vi "Example Configuration.vi"() -> ()   [LabVIEW 2013]
uses:
  C:/tf/play/labview/Tinkerforge.dll
panel:
  in  "uid":string="6dKCNw"
  in  "port":i32=4223
  in  "host":string="localhost"
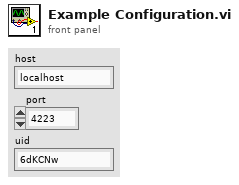
[diagram p1: front panel]
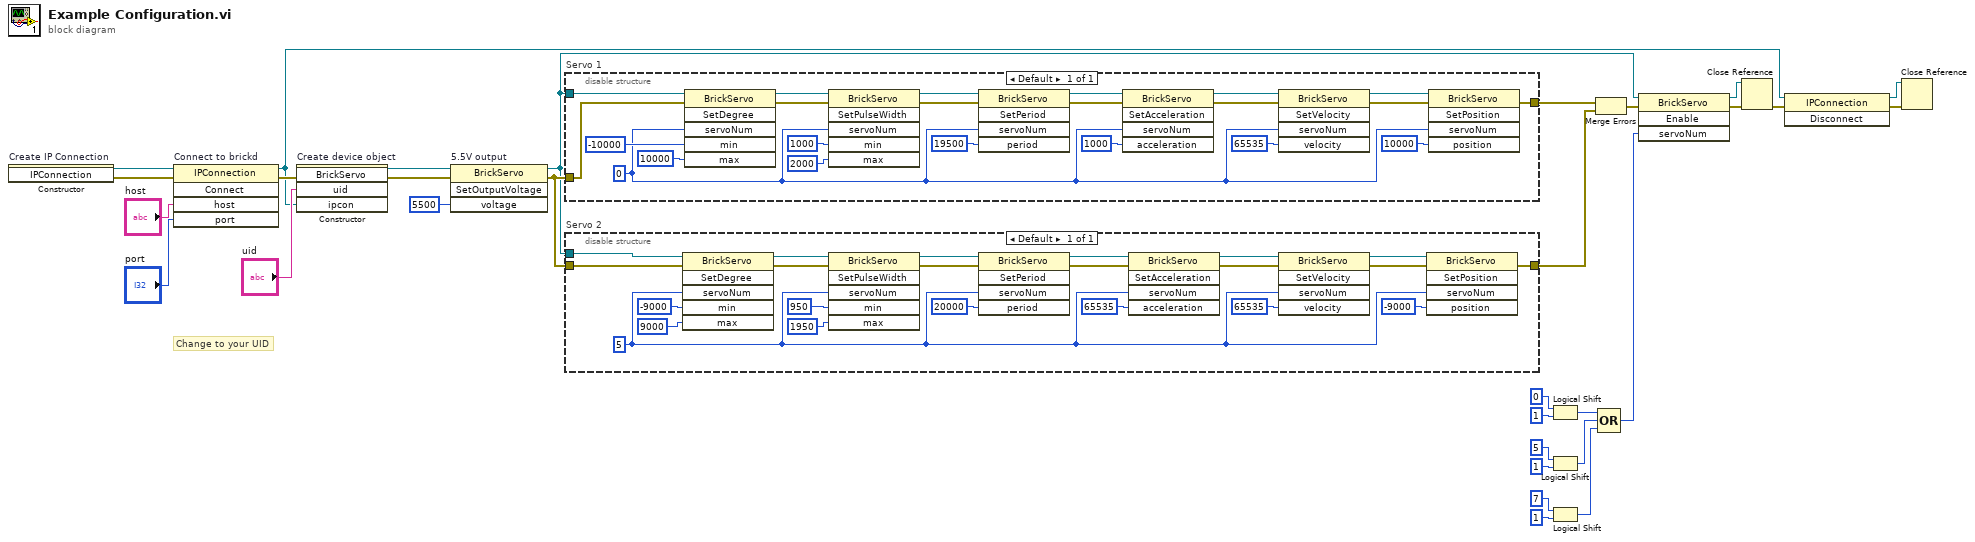
[diagram p0: block diagram]
diagram:
  # "Change to your UID"
  n1 = constructor on="Create IP Connection" class="IPConnection"() -> (reference out=w30:refnum<k24>, error out=w1:errorcluster)  [unwired: 3 in, 1 out]
  n2 = invoke on="Connect to brickd" class="IPConnection" method="Connect"(reference=w30, error in=w1, "host"="host", "port"="port") -> (reference out=w21:refnum<k24>, error out=w26:errorcluster)  [unwired: 1 in, 3 out]
  n3 = constructor on="Create device object" class="BrickServo"(error in=w26, "uid"="uid", "ipcon"=w21) -> (reference out=w24:refnum<k24>, error out=w25:errorcluster)  [unwired: 2 in, 3 out]
  n4 = invoke on="5.5V output" class="BrickServo" method="SetOutputVoltage"(reference=w24, error in=w25, "voltage"=5500 ("current")) -> (reference out=w15:refnum<k24>, error out=w18:errorcluster)  [unwired: 1 in, 2 out]
  n5 = disable-structure "Servo 1" shown="Default" {
    disable-tunnel: w15 -> [w50]
    disable-tunnel: w18 -> [w49]
    disable-tunnel: [w38] -> w16
    frame Enabled {
      w37 = u8 0 ("mode")
      n6 = invoke class="BrickServo" method="SetDegree"(reference=w50, error in=w49, "servoNum"=w37, "min"=i16 -10000, "max"=i16 10000) -> (reference out=w46:refnum<k24>, error out=w48:errorcluster)  [unwired: 1 in, 4 out]
      n7 = invoke class="BrickServo" method="SetPulseWidth"(reference=w46, error in=w48, "servoNum"=w37, "min"=1000, "max"=2000) -> (reference out=w45:refnum<k24>, error out=w47:errorcluster)  [unwired: 1 in, 4 out]
      n8 = invoke class="BrickServo" method="SetPeriod"(reference=w45, error in=w47, "servoNum"=w37, "period"=19500) -> (reference out=w43:refnum<k24>, error out=w44:errorcluster)  [unwired: 1 in, 3 out]
      n9 = invoke class="BrickServo" method="SetAcceleration"(reference=w43, error in=w44, "servoNum"=w37, "acceleration"=1000) -> (reference out=w41:refnum<k24>, error out=w42:errorcluster)  [unwired: 1 in, 3 out]
      n10 = invoke class="BrickServo" method="SetVelocity"(reference=w41, error in=w42, "servoNum"=w37, "velocity"=65535 ("acceleration")) -> (reference out=w39:refnum<k24>, error out=w40:errorcluster)  [unwired: 1 in, 3 out]
      n11 = invoke class="BrickServo" method="SetPosition"(reference=w39, error in=w40, "servoNum"=w37, "position"=i16 10000) -> (error out=w38:errorcluster)  [unwired: 1 in, 4 out]
    }
  }
  n12 = disable-structure "Servo 2" shown="Default" {
    disable-tunnel: w18 -> [w72]
    disable-tunnel: [w61] -> w17
    disable-tunnel: w15 -> [w59]
    frame Enabled {
      w60 = u8 5 ("mode")
      n13 = invoke class="BrickServo" method="SetDegree"(reference=w59, error in=w72, "servoNum"=w60, "min"=i16 -9000, "max"=i16 9000) -> (reference out=w69:refnum<k24>, error out=w71:errorcluster)  [unwired: 1 in, 4 out]
      n14 = invoke class="BrickServo" method="SetPulseWidth"(reference=w69, error in=w71, "servoNum"=w60, "min"=950, "max"=1950) -> (reference out=w68:refnum<k24>, error out=w70:errorcluster)  [unwired: 1 in, 4 out]
      n15 = invoke class="BrickServo" method="SetPeriod"(reference=w68, error in=w70, "servoNum"=w60, "period"=20000) -> (reference out=w66:refnum<k24>, error out=w67:errorcluster)  [unwired: 1 in, 3 out]
      n16 = invoke class="BrickServo" method="SetAcceleration"(reference=w66, error in=w67, "servoNum"=w60, "acceleration"=65535) -> (reference out=w64:refnum<k24>, error out=w65:errorcluster)  [unwired: 1 in, 3 out]
      n17 = invoke class="BrickServo" method="SetVelocity"(reference=w64, error in=w65, "servoNum"=w60, "velocity"=65535) -> (reference out=w62:refnum<k24>, error out=w63:errorcluster)  [unwired: 1 in, 3 out]
      n18 = invoke class="BrickServo" method="SetPosition"(reference=w62, error in=w63, "servoNum"=w60, "position"=i16 -9000) -> (error out=w61:errorcluster)  [unwired: 1 in, 4 out]
    }
  }
  n19 = Logical Shift(y=u8 0, x=u8 1) -> (x << y=w7:u8)
  n20 = Logical Shift(y=u8 5, x=u8 1) -> (x << y=w6:u8)
  n21 = Logical Shift(y=u8 7, x=u8 1) -> (x << y=w2:u8)
  n22 = Merge Errors(w16, w17) -> (w12:errorcluster)
  n23 = Compound Arithmetic op=OR(w7, w6, w2) -> (w5:u8)
  n24 = invoke class="BrickServo" method="Enable"(reference=w15, error in=w12, "servoNum"=w5) -> (reference out=w14:refnum<k24>, error out=w13:errorcluster)  [unwired: 1 in, 2 out]
  n25 = Close Reference(reference=w14, error in (no error)=w13) -> (error out=w23:errorcluster)
  n26 = invoke class="IPConnection" method="Disconnect"(reference=w21, error in=w23) -> (reference out=w20:refnum<k24>, error out=w22:errorcluster)  [unwired: 1 in, 1 out]
  n27 = Close Reference(reference=w20, error in (no error)=w22) -> ()  [unwired: 1 out]
